vi "RobotDriveOpen6MotorWithTalonSRX.vi"(0 "Left Motor 1":u8=255, 1 "Left Motor 2":u8=255, 2 "Left Motor 3":u8=255, 3 "Right Motor 1":u8=255, 4 "Right Motor 2":u8=255, 5 "Right Motor 3":u8=255, 7 "error in (no error)":errorcluster, 8 "Left Motor 1 Inverted":bool, 9 "Right Motor 1 Inverted":bool, 10 "Left Motor 2 Inverted":bool, 11 "Right Motor 2 Inverted":bool, 12 "Left Motor 3 Inverted":bool, 13 "Right Motor 3 Inverted":bool) -> (20 "RobotDriveDevRef":T1={"DevStatus"={"status"=FALSE, "code"=0, "source"=""}, "Motors[]"=[], "Square Inputs"=FALSE, "Max Output"=1.0}, 27 "error out":errorcluster)   [LabVIEW 2017, in "ArgosLib.lvlib"]
doc: "Opens a reference to the robot drive for a two-, four-, or six-motor robot using Talon SR motor controllers connected via CAN bus.\n\nFor 2-motor drive, connect Left Motor 1 and Right Motor 1.\nFor 4-motor drive, connect Left Motor 2 and Right Motor 2 in addition to the 2-motor drive connections.\nFor 6-motor drive, connect Left Motor 3 and Right Motor 3 in addition to the 4-motor drive connections.\n\nInversions are optional and are set to false if disconnected.\n\nThis software is licensed. Open the labview\\readme\\WPI Robotics Library Open Source License.txt file for more information."
uses:
  ArgosLib.lvlib
  <vilib>/Rock Robotics/WPI/RobotDrive/WPI_RobotDriveDevRef.ctl
  <vilib>/Rock Robotics/WPI/MotorControl/WPI_MotorControlDeviceRef.ctl
  <vilib>/Rock Robotics/WPI/MotorControl/WPI_MotorControlType.ctl
  <vilib>/Rock Robotics/SystemInterfaces/DIO/FPGA_DIOPWMChannel.ctl
  <vilib>/Rock Robotics/WPI/PWM/WPI_PWMDeadband.ctl
  <vilib>/Rock Robotics/SystemInterfaces/DIO/FPGA_DIOChannel.ctl
  <vilib>/Rock Robotics/WPI/SafetyOutput/WPI_SafetyOutputConfigMenu.ctl
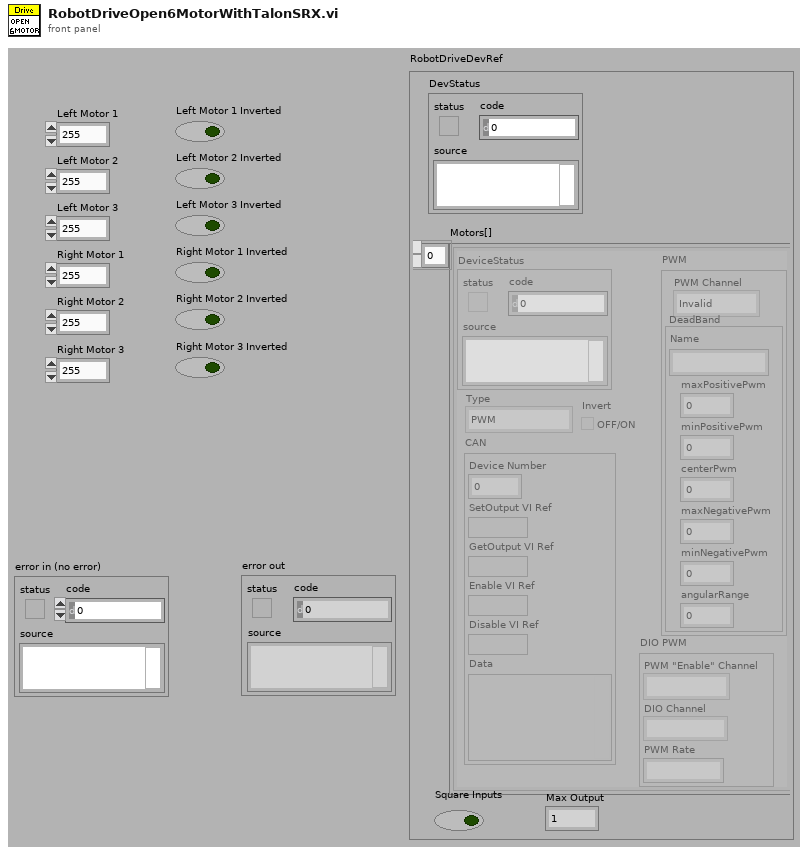
[diagram p1: front panel]
types:
  T1 = typedef "WPI_RobotDriveDevRef.ctl" = cluster{"DevStatus":errorcluster, "Motors[]":T2[], "Square Inputs":bool, "Max Output":dbl}
  T2 = typedef "WPI_MotorControlDeviceRef.ctl" = cluster{"DeviceStatus":errorcluster, "Type":T3, "PWM":cluster{"PWM Channel":T4, "DeadBand":T5}, "CAN":cluster{"Device Number":u8, "SetOutput VI Ref":variant, "GetOutput VI Ref":variant, "Enable VI Ref":variant, "Disable VI Ref":variant, "Data":variant}, "Invert":bool, "DIO PWM":cluster{"PWM \"Enable\" Channel":T4, "DIOChannel":T6, "PWM Rate":dbl}}
  T3 = typedef "WPI_MotorControlType.ctl" = enum16{"PWM", "CAN", "DIO PWM"}
  T4 = typedef "FPGA_DIOPWMChannel.ctl" = enum8{"PWM 0", "PWM 1", "PWM 2", "PWM 3", "PWM 4", "PWM 5", "PWM 6", "PWM 7", "PWM 8", "PWM 9", "PWM MXP 0", "PWM MXP 1", "PWM MXP 2", "PWM MXP 3", "PWM MXP 4", "PWM MXP 5", "PWM MXP 6", "PWM MXP 7", "PWM MXP 8", "PWM MXP 9", "Invalid"}
  T5 = typedef "WPI_PWMDeadband.ctl" = cluster{"Name":string, "maxPositivePwm":i32, "minPositivePwm":i32, "centerPwm":i32, "maxNegativePwm":i32, "minNegativePwm":i32, "angularRange":u16}
  T6 = typedef "FPGA_DIOChannel.ctl" = enum8{"DIO 0", "DIO 1", "DIO 2", "DIO 3", "DIO 4", "DIO 5", "DIO 6", "DIO 7", "DIO 8", "DIO 9", "DIO MXP 0", "DIO MXP 1", "DIO MXP 2", "DIO MXP 3", "DIO MXP 4", "DIO MXP 5", "DIO MXP 6", "DIO MXP 7", "DIO MXP 8", "DIO MXP 9", "DIO MXP 10", "DIO MXP 11", "DIO MXP 12", "DIO MXP 13", "DIO MXP 14", "DIO MXP 15", "SPI Port CS1", "SPI Port CS2", "SPI Port CS3", "SPI Port MISO", "SPI Port MOSI", "Invalid"}
  T7 = typedef "WPI_SafetyOutputConfigMenu.ctl" = enum16{"Enable", "Disable"}
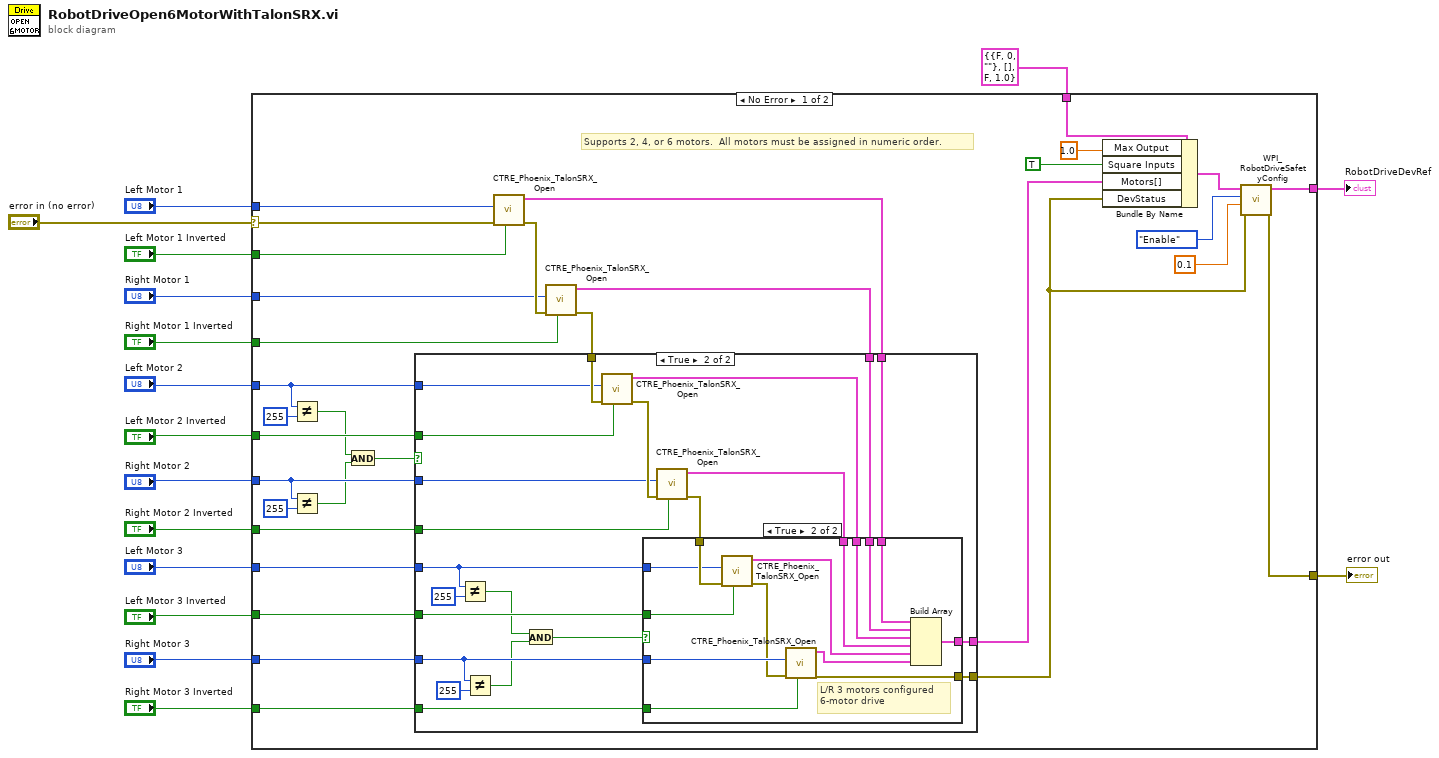
[diagram p0: block diagram]
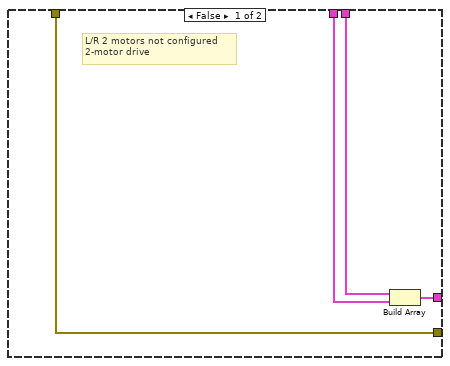
[diagram p2: hidden frame]
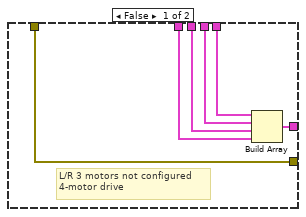
[diagram p3: hidden frame]
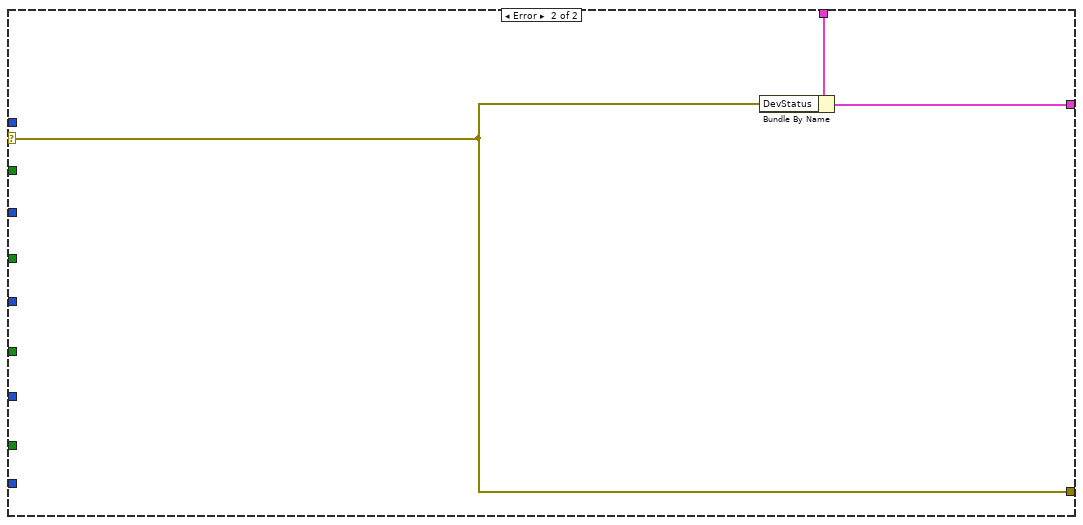
[diagram p4: hidden frame]
diagram:
  n1 = case shown="No Error" "error in (no error)" {
    selector: "error in (no error)" -> [w27 w95]
    tunnel: [w37 w96] -> w16
    tunnel: T1 {"DevStatus"={"status"=FALSE, "code"=0, "source"=""}, "Motors[]"=[], "Square Inputs"=FALSE, "Max Output"=1.0} ("RobotDriveDevRef") -> [w48 w97]
    tunnel: "Left Motor 1 Inverted" -> [w44 _]
    tunnel: "Right Motor 1 Inverted" -> [w43 _]
    tunnel: "Right Motor 2 Inverted" -> [w41 _]
    tunnel: "Left Motor 2 Inverted" -> [w42 _]
    tunnel: [w38 w95] -> w9
    tunnel: "Left Motor 3 Inverted" -> [w34 _]
    tunnel: "Right Motor 3 Inverted" -> [w33 _]
    tunnel: "Left Motor 1" -> [w31 _]
    tunnel: "Right Motor 1" -> [w30 _]
    tunnel: "Left Motor 2" -> [w26 _]
    tunnel: "Right Motor 2" -> [w23 _]
    tunnel: "Left Motor 3" -> [w29 _]
    tunnel: "Right Motor 3" -> [w28 _]
    frame No Error {
      # "Supports 2, 4, or 6 motors.  All motors must be assigned in numeric order."
      n2 = Not Equal?(x=w26, y=u8 255) -> (x != y?=w22:bool)
      n3 = Not Equal?(x=w23, y=u8 255) -> (x != y?=w21:bool)
      n4 = And(x=w22, y=w21) -> (x .and. y?=w20:bool)
      n5 = call <vilib>:"CTRE_Phoenix_TalonSRX_Open.vi"("Invert"=w44, "error in"=w27, "Device Number"=w31) -> ("error out"=w45:errorcluster, "CAN Talon SRX Ref"=w18:T2)  [unwired: 7 in]
      n6 = call <vilib>:"CTRE_Phoenix_TalonSRX_Open.vi"("Invert"=w43, "error in"=w45, "Device Number"=w30) -> ("error out"=w46:errorcluster, "CAN Talon SRX Ref"=w17:T2)  [unwired: 7 in]
      n7 = case shown="True" w20 {
        tunnel: w46 -> [w52 w73]
        tunnel: w42 -> [_ w72]
        tunnel: w41 -> [_ w71]
        tunnel: w34 -> [_ w69]
        tunnel: w33 -> [_ w68]
        tunnel: [w52 w67] -> w32
        tunnel: w29 -> [_ w61]
        tunnel: w28 -> [_ w62]
        tunnel: w26 -> [_ w66]
        tunnel: w23 -> [_ w65]
        tunnel: [w51 w57] -> w19
        tunnel: w18 -> [w50 w56]
        tunnel: w17 -> [w49 w55]
        frame False {
          # "L/R 2 motors not configured\n2-motor drive"
          n8 = Build Array(w50, w49) -> (w51:T2[])
        }
        frame True {
          n9 = Not Equal?(x=w61, y=u8 255) -> (x != y?=w59:bool)
          n10 = Not Equal?(x=w62, y=u8 255) -> (x != y?=w58:bool)
          n11 = And(x=w59, y=w58) -> (x .and. y?=w60:bool)
          n12 = call <vilib>:"CTRE_Phoenix_TalonSRX_Open.vi"("Invert"=w72, "error in"=w73, "Device Number"=w66) -> ("error out"=w74:errorcluster, "CAN Talon SRX Ref"=w54:T2)  [unwired: 7 in]
          n13 = call <vilib>:"CTRE_Phoenix_TalonSRX_Open.vi"("Invert"=w71, "error in"=w74, "Device Number"=w65) -> ("error out"=w70:errorcluster, "CAN Talon SRX Ref"=w53:T2)  [unwired: 7 in]
          n14 = case shown="True" w60 {
            tunnel: w70 -> [w80 w94]
            tunnel: w69 -> [_ w93]
            tunnel: w68 -> [_ w92]
            tunnel: [w80 w91] -> w67
            tunnel: w61 -> [_ w90]
            tunnel: w62 -> [_ w89]
            tunnel: [w79 w87] -> w57
            tunnel: w56 -> [w78 w86]
            tunnel: w55 -> [w77 w85]
            tunnel: w54 -> [w76 w84]
            tunnel: w53 -> [w75 w83]
            frame False {
              # "L/R 3 motors not configured\n4-motor drive"
              n15 = Build Array(w78, w77, w76, w75) -> (w79:T2[])
            }
            frame True {
              # "L/R 3 motors configured\n6-motor drive"
              n16 = call <vilib>:"CTRE_Phoenix_TalonSRX_Open.vi"("Invert"=w93, "error in"=w94, "Device Number"=w90) -> ("error out"=w88:errorcluster, "CAN Talon SRX Ref"=w82:T2)  [unwired: 7 in]
              n17 = call <vilib>:"CTRE_Phoenix_TalonSRX_Open.vi"("Invert"=w92, "error in"=w88, "Device Number"=w89) -> ("error out"=w91:errorcluster, "CAN Talon SRX Ref"=w81:T2)  [unwired: 7 in]
              n18 = Build Array(w86, w85, w84, w83, w82, w81) -> (w87:T2[])
            }
          }
        }
      }
      n19 = Bundle By Name(cluster=w48, "Max Output"=1.0, "Square Inputs"=TRUE ("DestroyPWM?"), "Motors[]"=w19, "DevStatus"=w32) -> (w39:T1)
      n20 = call <vilib>:"WPI_RobotDriveSafetyConfig.vi"("error in (no error)"=w32, "timeout (s)"=0.1, "mode"=WPI_SafetyOutputConfigMenu."Enable", "RobotDriveDevRef"=w39) -> ("error out"=w38:errorcluster, "RobotDriveDevRef"=w37:T1)  [unwired: 6 out]
    }
    frame Error {
      n21 = Bundle By Name(cluster=w97, "DevStatus"=w95) -> (w96:T1)
    }
  }
  "RobotDriveDevRef" <- w16
  "error out" <- w9
